vi "Semi Auto Elevator Loop.vi"() -> (2 "Elevator Power":dbl)   [LabVIEW 2017]
uses:
  Robot Global Data.vi
  Common Code/Elevator State.ctl
  <vilib>/addons/control/pid/NI_PID_pid.lvlib
  <vilib>/addons/control/pid/pid.llb/PID (DBL).vi
panel:
  out "Finished?":bool
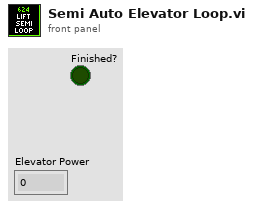
[diagram p1: front panel]
types:
  T1 = typedef "Elevator State.ctl" = enum16{"Idle", "Ground", "Mid", "Scale", "Switch"}
  T2 = typedef "Dashboard Control Data.ctl" = cluster{"Drivetrain Settings Cluster":T3, "Intake Presets":T5, "Elevator Settings Cluster":T6}
  T3 = typedef "Drivetrain Settings Clustr.ctl" = cluster{"Gyro Steer PID Gains":T4, "Distance Drive PID Gains":T4, "Drive Tolerance":dbl, "Gyro Tolerance":dbl, "Gyro Output":dbl, "Distance Output":dbl, "Y Power Multiplier":dbl, "Turn Power Multiplier":dbl, "Creep Rate":dbl, "Constant Power":bool, "DT Mode Modifier":enum16{"None, Default", "Cube", "Square"}, "Left Encoder Tick Constant":dbl, "Right Encoder Tick Constant":dbl, "Shift Speed":dbl}
  T4 = typedef "PID Gains Cluster.ctl" = cluster{"Integral Time":dbl, "Proportional Gain":dbl, "Derivative Time":dbl}
  T5 = typedef "Intake Presets.ctl" = cluster{"Idle Angle":dbl, "Mid Angle":dbl, "Low Angle":dbl, "Outtake Power":dbl, "Intake Power":dbl, "Unstuck":dbl, "Angle Tolerance":dbl, "Max Angle":dbl, "Max Current":dbl, "Current Trip Time":dbl, "Reset Encoder?":bool, "Encoder Scale":dbl, "PID gains":cluster{"proportional gain (Kc)":dbl, "integral time (Ti, min)":dbl, "derivative time (Td, min)":dbl}, "output range":cluster{"output high":dbl, "output low":dbl}}
  T6 = typedef "Elevator Settings Cluster.ctl" = cluster{"Ground Height":dbl, "Switch Height":dbl, "Scale High Height ":dbl, "Scale Low Height":dbl, "Elevator PID Gains":T7, "Elevator Tolerance":dbl, "Reset Encoders":bool, "Encoder Scale":dbl, "Max Height":dbl, "Mid Height":dbl, "output range":cluster{"output high":dbl, "output low":dbl}}
  T7 = typedef "PID Gains.ctl" = cluster{"proportional gain (Kc)":dbl, "integral time (Ti, min)":dbl, "derivative time (Td, min)":dbl}
  T8 = typedef "Elevator Command Cluster.ctl" = cluster{"Elevator Mode":T9, "Elevator State":T1, "Manual Speed":dbl, "Reset Encoders":bool, "High?":bool}
  T9 = typedef "Elevator Mode.ctl" = enum16{"Semi Auto", "Manual", "Auto"}
  T10 = typedef "Elevator Status Cluster.ctl" = cluster{"Finished":bool, "Output":dbl, "Elevator State":T1, "Elevator Mode":T9, "Encoder Height":dbl, "Elevator Height":dbl, "At Bottom?":bool, "At Top?":bool}
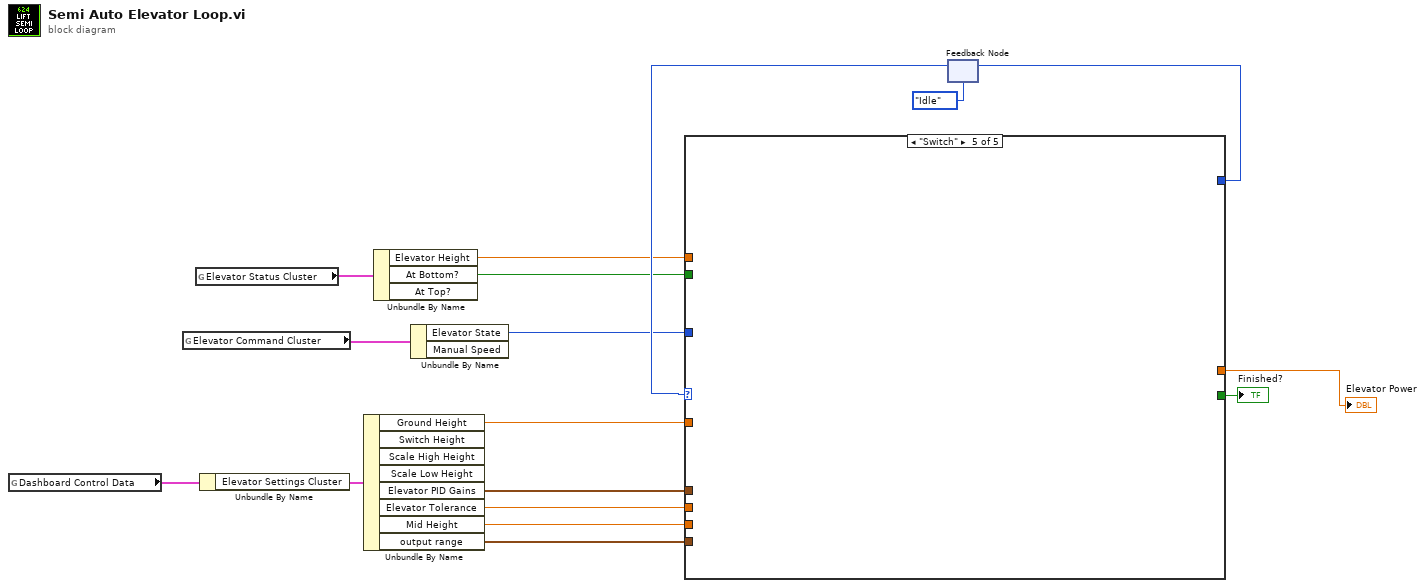
[diagram p0: block diagram]
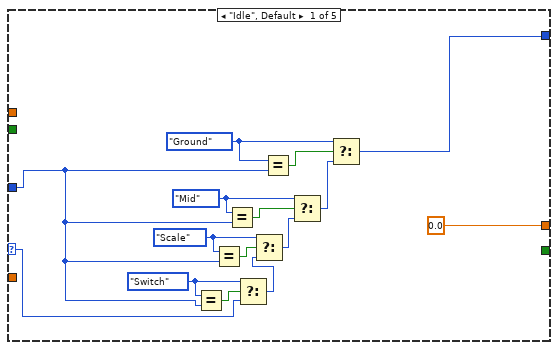
[diagram p2: hidden frame]
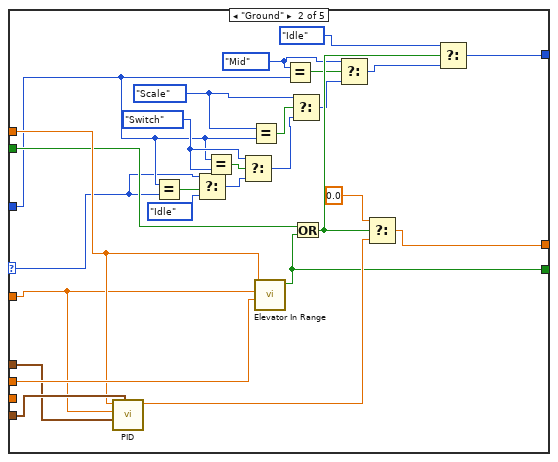
[diagram p3: hidden frame]
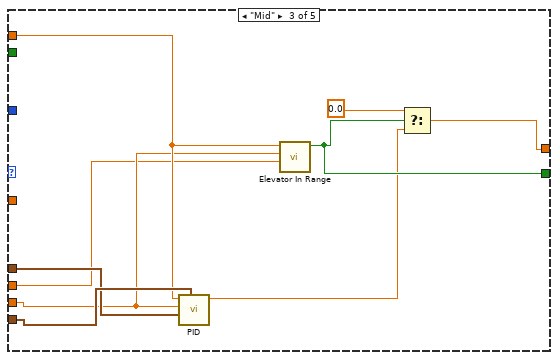
[diagram p4: hidden frame]
diagram:
  n1 = global read "Robot Global Data.vi" "Dashboard Control Data"() -> (w16:T2)
  n2 = global read "Robot Global Data.vi" "Elevator Command Cluster"() -> (w17:T8)
  n3 = global read "Robot Global Data.vi" "Elevator Status Cluster"() -> (w10:T10)
  n4 = Unbundle By Name(w16) -> ("Elevator Settings Cluster"=w15:T6)
  n5 = Unbundle By Name(w15) -> ("Ground Height"=w5:dbl, "Elevator PID Gains"=w3:T7, "Elevator Tolerance"=w4:dbl, "Mid Height"=w1:dbl, "output range"=w8:cluster{"output high":dbl, "output low":dbl})  [unwired: 3 out]
  n6 = Unbundle By Name(w10) -> ("Elevator Height"=w7:dbl, "At Bottom?"=w6:bool)  [unwired: 1 out]
  n7 = Unbundle By Name(w17) -> ("Elevator State"=w12:T1)  [unwired: 1 out]
  n8 = feedback #1(Elevator_State."Idle" ("Elevator State")) -> (w13:T1)
  n9 = case shown="\"Switch\"" w13 {
    selector: w13 -> [w19 w36 _ _ _]
    tunnel: w12 -> [w26 w38 _ _ _]
    tunnel: [0.0 w52 w61 _ _] -> w11
    tunnel: [w18 w33 _ _ _] -> w9
    tunnel: w8 -> [_ w59 w68 _ _]
    tunnel: w7 -> [_ w57 w66 _ _]
    tunnel: w6 -> [_ w45 _ _ _]
    tunnel: w5 -> [_ w56 _ _ _]
    tunnel: w4 -> [_ w58 w64 _ _]
    tunnel: w3 -> [_ w53 w67 _ _]
    tunnel: [_ w51 w63 _ _] -> w2
    tunnel: w1 -> [_ _ w65 _ _]
    frame "Idle", Default {
      w25 = Elevator_State."Switch" ("Elevator State")
      w24 = Elevator_State."Scale" ("Elevator State")
      w23 = Elevator_State."Mid" ("Elevator State")
      w30 = Elevator_State."Ground" ("Elevator State")
      n10 = Equal?(x=w25, y=w26) -> (x = y?=w27:bool)
      n11 = Equal?(x=w24, y=w26) -> (x = y?=w28:bool)
      n12 = Equal?(x=w23, y=w26) -> (x = y?=w29:bool)
      n13 = Select(t=w25, s=w27, f=w19) -> (s? t:f=w20:T1)
      n14 = Select(t=w24, s=w28, f=w20) -> (s? t:f=w21:T1)
      n15 = Equal?(x=w30, y=w26) -> (x = y?=w31:bool)
      n16 = Select(t=w23, s=w29, f=w21) -> (s? t:f=w22:T1)
      n17 = Select(t=w30, s=w31, f=w22) -> (s? t:f=w18:T1)
    }
    frame "Ground" {
      w40 = Elevator_State."Switch" ("Elevator State")
      w43 = Elevator_State."Scale" ("Elevator State")
      w47 = Elevator_State."Mid" ("Elevator State")
      n18 = call-poly <vilib>:"PID.vi"("output range"=w59, "PID gains"=w53, "process variable"=w56, "setpoint"=w57) -> ("output"=w54:dbl)  [unwired: 6 in, 1 out]
      n19 = Equal?(x=w38, y=w36) -> (x = y?=w37:bool)
      n20 = Select(t=w36, s=w37, f=Elevator_State."Idle" ("Elevator State")) -> (s? t:f=w35:T1)
      n21 = Equal?(x=w38, y=w40) -> (x = y?=w41:bool)
      n22 = Select(t=w40, s=w41, f=w35) -> (s? t:f=w39:T1)
      n23 = Equal?(x=w43, y=w38) -> (x = y?=w42:bool)
      n24 = call "Elevator In Range.vi"("Height Tolerance"=w58, "Target Height"=w56, "Actual Height"=w57) -> ("In Range"=w51:bool)  [unwired: 8 in]
      n25 = Equal?(x=w47, y=w38) -> (x = y?=w48:bool)
      n26 = Select(t=w43, s=w42, f=w39) -> (s? t:f=w44:T1)
      n27 = Or(x=w45, y=w51) -> (x .or. y?=w50:bool)
      n28 = Select(t=w47, s=w48, f=w44) -> (s? t:f=w46:T1)
      n29 = Select(t=0.0, s=w50, f=w54) -> (s? t:f=w52:dbl)
      n30 = Select(t=Elevator_State."Idle" ("Elevator State"), s=w50, f=w46) -> (s? t:f=w33:T1)
    }
    frame "Mid" {
      n31 = call-poly <vilib>:"PID.vi"("output range"=w68, "PID gains"=w67, "process variable"=w65, "setpoint"=w66) -> ("output"=w60:dbl)  [unwired: 6 in, 1 out]
      n32 = call "Elevator In Range.vi"("Height Tolerance"=w64, "Target Height"=w65, "Actual Height"=w66) -> ("In Range"=w63:bool)  [unwired: 8 in]
      n33 = Select(t=0.0, s=w63, f=w60) -> (s? t:f=w61:dbl)
    }
    frame "Scale" {
    }
    frame "Switch" {
    }
  }
  "Elevator Power" <- w11
  "Finished?" <- w2
  n34 = feedback-in #1(w9) -> ()
